vi "LVClass_DataClient GetBoolean.vi"(0 "DataClient in":refnum<class "DataClient.lvclass">, 5 "name":string, 11 "error in (no error)":errorcluster) -> (4 "DataClient out":refnum<class "DataClient.lvclass">, 8 "Value":bool, 10 "data_unique_id":i32, 15 "error out":errorcluster)   [LabVIEW 2020, in "DataClient.lvclass"]
doc: "Boolean getter.\n\n<B>clientIn</B> : Client object.\n<B>clientOut</B> : Client object.\n<B>data_name</B> : Data name.\n<B>data</B> : Data content.\n<B>data_id</B> : Data content id."
uses:
  DataClient.lvclass
  DataClient.lvclass/DataClient.ctl
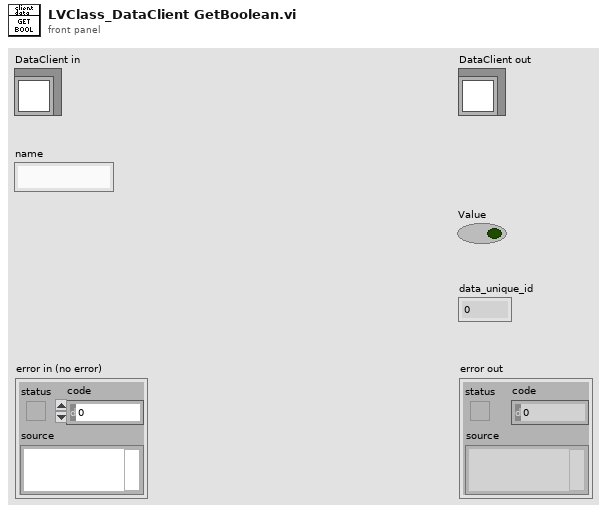
[diagram p1: front panel]
types:
  T1 = typedef "ClassID.ctl" = i64
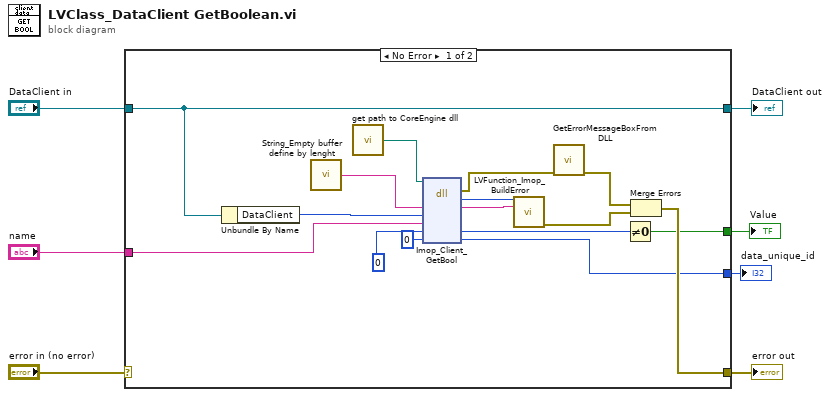
[diagram p0: block diagram]
diagram:
  n1 = case shown="No Error" "error in (no error)" {
    selector: "error in (no error)" -> [_ w25]
    tunnel: [w14 w25] -> w6
    tunnel: [w15 w24] -> w4
    tunnel: "DataClient in" -> [w15 w24]
    tunnel: [w8 _] -> w3
    tunnel: "name" -> [w13 _]
    tunnel: [w11 _] -> w1
    frame No Error {
      n2 = Unbundle By Name(w15) -> ("DataClient"=w18:T1)
      n3 = call "String_Empty buffer define by lenght.vi"() -> ("Empty buffer"=w21:string)  [unwired: 1 in]
      n4 = call "get path to CoreEngine dll.vi"() -> ("path to wavekit library"=w20:path)  [unwired: 14 in, 1 out]
      n5 = dll-call lib="D:/soft/HASO_v3/SVN_trunk/ImOpCoreEngine4_LV2011/DLLs/c_interface_vc100.dll" fn="Imop_Client_GetBool"(path in=w20, "message"=w21, "client"=w18, "name"=w13, "bool"=u8 0, "data_id"=0) -> (error out=w19:errorcluster, "return type"=w23:i32, "message"=w22:string, "bool"=w9:u8, "data_id"=w11:i32)  [unwired: 4 in, 1 out]
      n6 = call "LVFunction_Imop_BuildError.vi"("code"=w23, "String to Prepend to source (\"\")"=w22) -> ("error out"=w16:errorcluster)  [unwired: 13 in]
      n7 = call "GetErrorMessageBoxFromDLL.vi"("error IN"=w19) -> ("error OUT"=w17:errorcluster)  [unwired: 10 in]
      n8 = Not Equal To 0?(x=w9) -> (x != 0?=w8:bool)
      n9 = Merge Errors(w17, w16) -> (w14:errorcluster)
    }
    frame Error {
    }
  }
  "error out" <- w6
  "DataClient out" <- w4
  "Value" <- w3
  "data_unique_id" <- w1
